vi "Get Path Regex.vi"(8 "error in (no error)":errorcluster, 11 "Pending Submissions in":refnum<class "Admin Info.lvclass">) -> (0 "error out":errorcluster, 2 "Path Regex":string, 3 "Pending Submissions out":refnum<class "Admin Info.lvclass">)   [LabVIEW 2020, in "Summer of LabVIEW.lvlib" / "Admin Info.lvclass"]
uses:
  Admin Info.lvclass
  Admin Info.lvclass/Admin Info.ctl
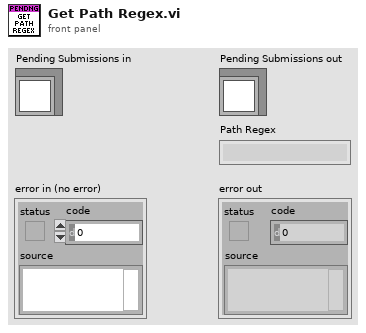
[diagram p1: front panel]
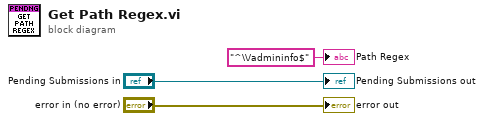
[diagram p0: block diagram]
diagram:
  "error out" <- "error in (no error)"
  "Pending Submissions out" <- "Pending Submissions in"
  "Path Regex" <- "^\\/admininfo$" ("Path Regex")
